vi "Search Home.vi"(8 "error in (no error)":errorcluster, 9 "Home Mode":i32=1, 10 "Axis":i32=1, 11 "Simulated in":refnum<class "Simulated-TS.lvclass">) -> (0 "error out":errorcluster, 3 "Simulated out":refnum<class "Simulated-TS.lvclass">)   [LabVIEW 2019, in "Simulated-TS.lvclass"]
uses:
  Simulated-TS.lvclass
  Simulated-TS.lvclass/Simulated-TS.ctl
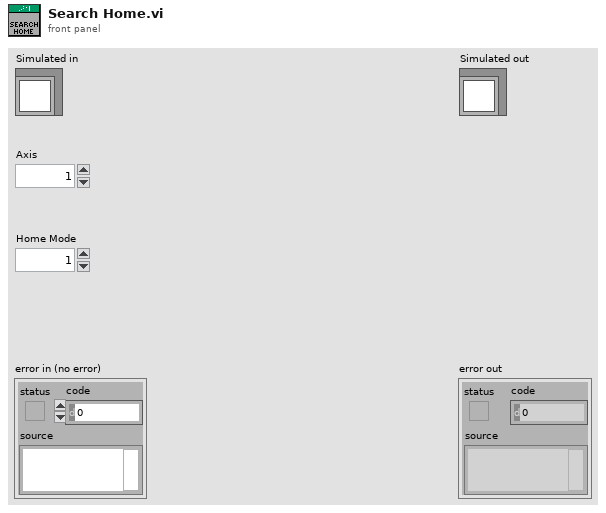
[diagram p1: front panel]
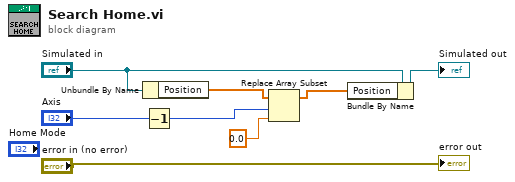
[diagram p0: block diagram]
diagram:
  n1 = Unbundle By Name("Simulated in") -> ("Position"=w5:dbl[])
  n2 = Decrement(x="Axis") -> (x-1=w3:i32)
  n3 = Replace Array Subset(array=w5, new element=0.0 ("new element/subarray"), index=w3) -> (w1:dbl[])
  n4 = Bundle By Name(cluster="Simulated in", "Position"=w1) -> (→"Simulated out":refnum<class "Simulated-TS.lvclass">)
  "error out" <- "error in (no error)"
